vi "Configure test.vi"(6 "Assert VI Path":path, 7 "Existing Queue Elements":string, 8 "error in (no error)":errorcluster, 11 "Basic Str Ends With in":refnum<class "Str Ends With.lvclass">) -> (0 "error out":errorcluster, 3 "Basic Str Ends With out":refnum<class "Str Ends With.lvclass">)   [LabVIEW 2018, in "Str Ends With.lvclass"]
uses:
  Str Ends With.lvclass
  <vilib>/Utility/Data Type/Type Definitions/Data Type.ctl
  0d99fb3d-a7f6-45d6-b308-e2c02a3f7416.vi
  <vilib>/JDP Science/JSONtext/Find Item.vi
  0d99fb3d-a7f6-45d6-b308-e2c02a3f7416.vi/429c71c6-5139-4d85-8902-9291fb8fc611.vi
  0d99fb3d-a7f6-45d6-b308-e2c02a3f7416.vi/6b17c3a5-76c9-4440-a0a2-4599ec43e7c4.vi
  <vilib>/JDP Science/JSONtext/String Subset.vi
  Test Class String IDs.vi
  <vilib>/JDP Science/JSONtext/Parsing/Parse Full Path or Item Name.vi
  <vilib>/JDP Science/JSONtext/Offset/Find Item Locations by Path.vi
  <vilib>/JDP Science/JSONtext/JSON text to Variant.vi
  <vilib>/JDP Science/JSONtext/Variant to JSON Text.vi
  <vilib>/JDP Science/JSONtext/Set Item.vi
  String.lvclass
  Test.lvclass
  <vilib>/Utility/Data Type/NI_Data Type.lvlib
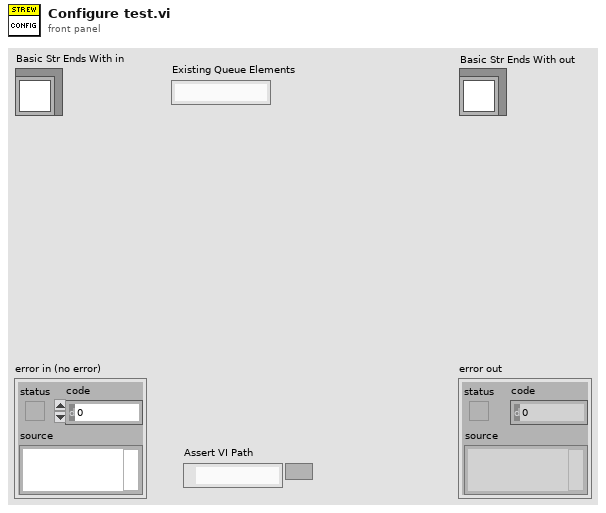
[diagram p1: front panel]
types:
  T1 = typedef "NI_Data Type.lvlib/Data Type.ctl" = enum8{"Invalid Type", "Void", "I8", "I16", "I32", "I64", "U8", "U16", "U32", "U64", "Single Float", "Double Float", "Extended Float", "Single Complex", "Double Complex", "Extended Complex", "Enum U8", "Enum U16", "Enum U32", "Enum U64", "Single Float With Unit", "Double Float With Unit", "Extended Float With Unit", "Single Complex with Unit", "Double Complex with Unit", "Extended Complex with Unit", "Boolean", "String", "Path", "Picture", "Tag", "Array", "Cluster", "Variant", "LV Variant", "Waveform", "Timestamp", "Digital Waveform", "Digital Data", "ExpressData", "Refnum", "External Data", "VI", "Poly VI", "LabVIEW Class Instance", "Fixed Point"}
  T2 = cluster{"Additional Data":string, "Comparison Value":string, "Invert?":string, "Assert Name":string, "Comment":string, "Default Failure Action":string, "Assert Build Timestamp":string, "Assert Builder User Name":string, "Data Type":string, "Assert VI Name":string, "Evaluation String":string}
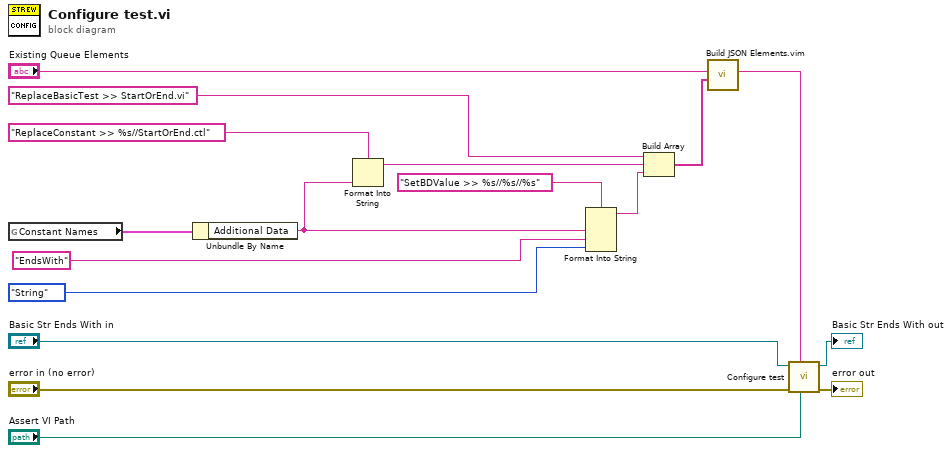
[diagram p0: block diagram]
diagram:
  n1 = global read "Test Class String IDs.vi" "Constant Names"() -> (w8:T2)
  n2 = Unbundle By Name(w8) -> ("Additional Data"=w7:string)
  n3 = Format Into String(format string="ReplaceConstant >> %s//StartOrEnd.ctl" ("Append Element(s)"), w7) -> (resulting string=w9:string)  [unwired: 2 in, 1 out]
  n4 = Format Into String(format string="SetBDValue >> %s//%s//%s", w7, "EndsWith" ("input 2"), Data_Type."String" ("input 3")) -> (resulting string=w11:string)  [unwired: 2 in, 1 out]
  n5 = Build Array("ReplaceBasicTest >> StartOrEnd.vi" ("Append Element(s)"), w9, w11) -> (w3:string[])
  n6 = call "Build JSON Elements.vim"("Append Element(s)"=w3, "JSON Elements in ({})"="Existing Queue Elements") -> ("JSON Elements out"=w1:string)  [unwired: 9 in]
  n7 = call-parent "Configure test.vi"("Assert VI Path"="Assert VI Path", "Existing Queue Elements"=w1, "error in (no error)"="error in (no error)", "Basic String in"="Basic Str Ends With in") -> ("error out"=→"error out":errorcluster, "Basic String out"=→"Basic Str Ends With out":refnum<class "Str Ends With.lvclass">)  [unwired: 6 in]
